vi "String to end-stop.vi"(8 "error in (no error)":errorcluster, 11 "String":string) -> (0 "error out":errorcluster, 3 "End-stop status":bool[](array[boolean]))   [LabVIEW 2020, in "Arduino-Adafruit stepper.lvlib"]
uses:
  Arduino-Adafruit stepper.lvlib
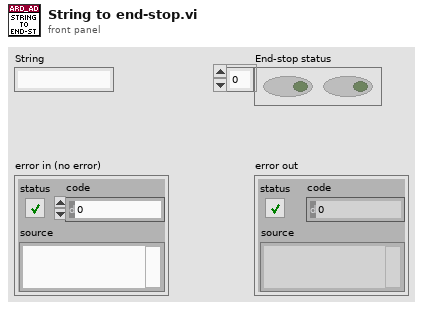
[diagram p1: front panel]
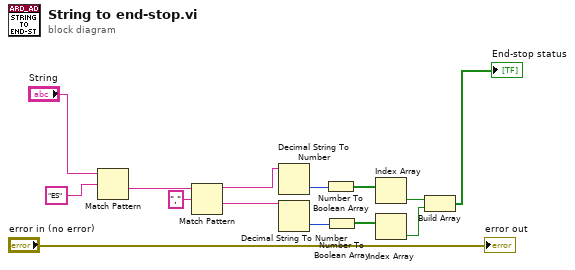
[diagram p0: block diagram]
diagram:
  n1 = Match Pattern(string="String", regular expression="ES") -> (after substring=w4:string)  [unwired: 1 in, 3 out]
  n2 = Match Pattern(string=w4, regular expression=",") -> (before substring=w5:string, after substring=w6:string)  [unwired: 1 in, 2 out]
  n3 = Decimal String To Number(string=w5) -> (number=w7:i32)  [unwired: 2 in, 1 out]
  n4 = Decimal String To Number(string=w6) -> (number=w8:i32)  [unwired: 2 in, 1 out]
  n5 = Number To Boolean Array(number=w7) -> (Boolean array=w9:bool[])
  n6 = Number To Boolean Array(number=w8) -> (Boolean array=w10:bool[])
  n7 = Index Array(array=w9) -> (element=w11:bool)  [unwired: 1 in]
  n8 = Index Array(array=w10) -> (element=w12:bool)  [unwired: 1 in]
  n9 = Build Array(w11, w12) -> (→"End-stop status":bool[])
  "error out" <- "error in (no error)"
